vi "listener_parameters_selector.vi"(6 "stations":T4, 11 "all_config_info_out":T1) -> (2 "listener port":u16, 3 "listener IP":string)   [LabVIEW 2020]
uses:
  station.ctl
  ini/typedef/PROXY_all_config_info.ctl
  ini/typedef/PROXY_main_ini_file.ctl
  queues/typedef/PROXY_queue_refnums.ctl
  queues/typedef/STATION_queue_element.ctl
  ST_SQL_sequence_state.ctl
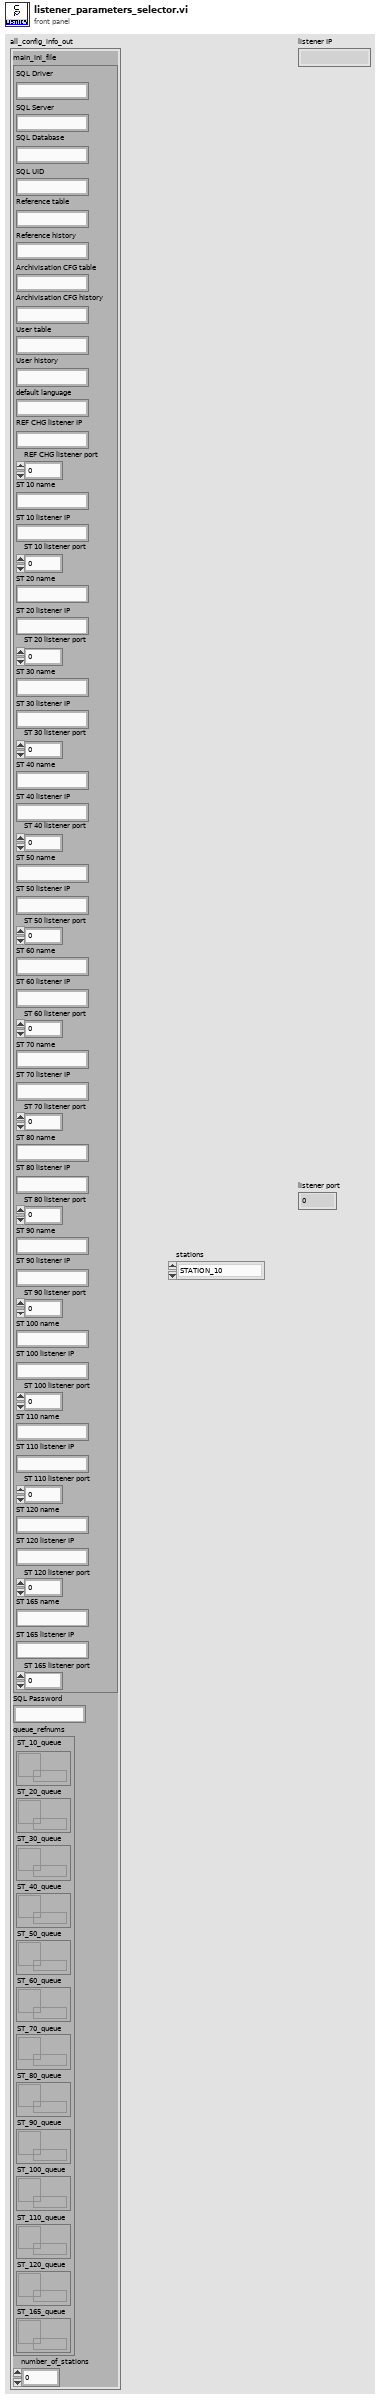
[diagram p1: front panel]
types:
  T1 = typedef "PROXY_all_config_info.ctl" = cluster{"main_ini_file":T2, "SQL Password":string, "queue_refnums":T3, "number_of_stations":i32}
  T2 = typedef "PROXY_main_ini_file.ctl" = cluster{"SQL Driver":string, "SQL Server":string, "SQL Database":string, "SQL UID":string, "Reference table":string, "Reference history":string, "Archivisation CFG table":string, "Archivisation CFG history":string, "User table":string, "User history":string, "default language":string, "REF CHG listener IP":string, "REF CHG listener port":u16, "ST 10 name":string, "ST 10 listener IP":string, "ST 10 listener port":u16, "ST 20 name":string, "ST 20 listener IP":string, "ST 20 listener port":u16, "ST 30 name":string, "ST 30 listener IP":string, "ST 30 listener port":u16, "ST 40 name":string, "ST 40 listener IP":string, "ST 40 listener port":u16, "ST 50 name":string, "ST 50 listener IP":string, "ST 50 listener port":u16, "ST 60 name":string, "ST 60 listener IP":string, "ST 60 listener port":u16, "ST 70 name":string, "ST 70 listener IP":string, "ST 70 listener port":u16, "ST 80 name":string, "ST 80 listener IP":string, "ST 80 listener port":u16, "ST 90 name":string, "ST 90 listener IP":string, "ST 90 listener port":u16, "ST 100 name":string, "ST 100 listener IP":string, "ST 100 listener port":u16, "ST 110 name":string, "ST 110 listener IP":string, "ST 110 listener port":u16, "ST 120 name":string, "ST 120 listener IP":string, "ST 120 listener port":u16, "ST 165 name":string, "ST 165 listener IP":string, "ST 165 listener port":u16}
  T3 = typedef "PROXY_queue_refnums.ctl" = cluster{"ST_10_queue":refnum<queue>, "ST_20_queue":refnum<queue>, "ST_30_queue":refnum<queue>, "ST_40_queue":refnum<queue>, "ST_50_queue":refnum<queue>, "ST_60_queue":refnum<queue>, "ST_70_queue":refnum<queue>, "ST_80_queue":refnum<queue>, "ST_90_queue":refnum<queue>, "ST_100_queue":refnum<queue>, "ST_110_queue":refnum<queue>, "ST_120_queue":refnum<queue>, "ST_165_queue":refnum<queue>}
  T4 = typedef "station.ctl" = enum16{"STATION_10", "STATION_20", "STATION_30", "STATION_40", "STATION_50", "STATION_60", "STATION_70", "STATION_80", "STATION_90", "STATION_100", "STATION_110", "STATION_120", "STATION_165", "MAIN"}
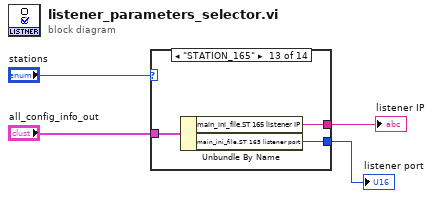
[diagram p0: block diagram]
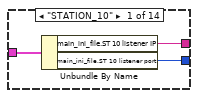
[diagram p2: hidden frame]
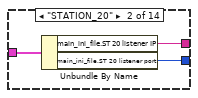
[diagram p3: hidden frame]
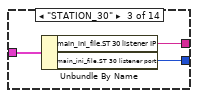
[diagram p4: hidden frame]
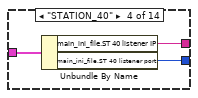
[diagram p5: hidden frame]
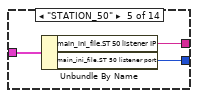
[diagram p6: hidden frame]
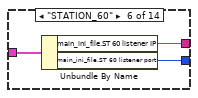
[diagram p7: hidden frame]
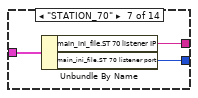
[diagram p8: hidden frame]
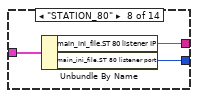
[diagram p9: hidden frame]
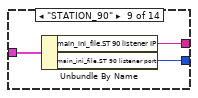
[diagram p10: hidden frame]
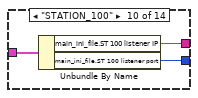
[diagram p11: hidden frame]
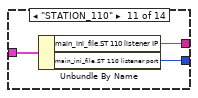
[diagram p12: hidden frame]
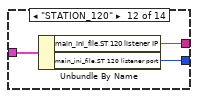
[diagram p13: hidden frame]
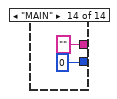
[diagram p14: hidden frame]
diagram:
  n1 = case shown="\"STATION_165\"" "stations" {
    tunnel: [w7 w10 w13 w16 w19 w22 w25 w28 w31 w34 w37 w40 w43 u16 0 ("ST30 listener port")] -> w1
    tunnel: [w6 w9 w12 w15 w18 w21 w24 w27 w30 w33 w36 w39 w42 "" ("ST30 listener IP")] -> w2
    tunnel: "all_config_info_out" -> [w5 w8 w11 w14 w17 w20 w23 w26 w29 w32 w35 w38 w41 _]
    frame "STATION_10" {
      n2 = Unbundle By Name(w5) -> ("main_ini_file.ST 10 listener IP"=w6:string, "main_ini_file.ST 10 listener port"=w7:u16)
    }
    frame "STATION_20" {
      n3 = Unbundle By Name(w8) -> ("main_ini_file.ST 20 listener IP"=w9:string, "main_ini_file.ST 20 listener port"=w10:u16)
    }
    frame "STATION_30" {
      n4 = Unbundle By Name(w11) -> ("main_ini_file.ST 30 listener IP"=w12:string, "main_ini_file.ST 30 listener port"=w13:u16)
    }
    frame "STATION_40" {
      n5 = Unbundle By Name(w14) -> ("main_ini_file.ST 40 listener IP"=w15:string, "main_ini_file.ST 40 listener port"=w16:u16)
    }
    frame "STATION_50" {
      n6 = Unbundle By Name(w17) -> ("main_ini_file.ST 50 listener IP"=w18:string, "main_ini_file.ST 50 listener port"=w19:u16)
    }
    frame "STATION_60" {
      n7 = Unbundle By Name(w20) -> ("main_ini_file.ST 60 listener IP"=w21:string, "main_ini_file.ST 60 listener port"=w22:u16)
    }
    frame "STATION_70" {
      n8 = Unbundle By Name(w23) -> ("main_ini_file.ST 70 listener IP"=w24:string, "main_ini_file.ST 70 listener port"=w25:u16)
    }
    frame "STATION_80" {
      n9 = Unbundle By Name(w26) -> ("main_ini_file.ST 80 listener IP"=w27:string, "main_ini_file.ST 80 listener port"=w28:u16)
    }
    frame "STATION_90" {
      n10 = Unbundle By Name(w29) -> ("main_ini_file.ST 90 listener IP"=w30:string, "main_ini_file.ST 90 listener port"=w31:u16)
    }
    frame "STATION_100" {
      n11 = Unbundle By Name(w32) -> ("main_ini_file.ST 100 listener IP"=w33:string, "main_ini_file.ST 100 listener port"=w34:u16)
    }
    frame "STATION_110" {
      n12 = Unbundle By Name(w35) -> ("main_ini_file.ST 110 listener IP"=w36:string, "main_ini_file.ST 110 listener port"=w37:u16)
    }
    frame "STATION_120" {
      n13 = Unbundle By Name(w38) -> ("main_ini_file.ST 120 listener IP"=w39:string, "main_ini_file.ST 120 listener port"=w40:u16)
    }
    frame "STATION_165" {
      n14 = Unbundle By Name(w41) -> ("main_ini_file.ST 165 listener IP"=w42:string, "main_ini_file.ST 165 listener port"=w43:u16)
    }
    frame "MAIN" {
    }
  }
  "listener IP" <- w2
  "listener port" <- w1
